vi "FileExplorer.vi"() -> ()   [LabVIEW 2010]
panel:
  in  "löschen":bool
  out "Numeric":i32
  out "error out 2":errorcluster
  out "filenames":string[](array[string])
  out "folder names":string[](array[string])
  out "error out":errorcluster
  in  "path":path
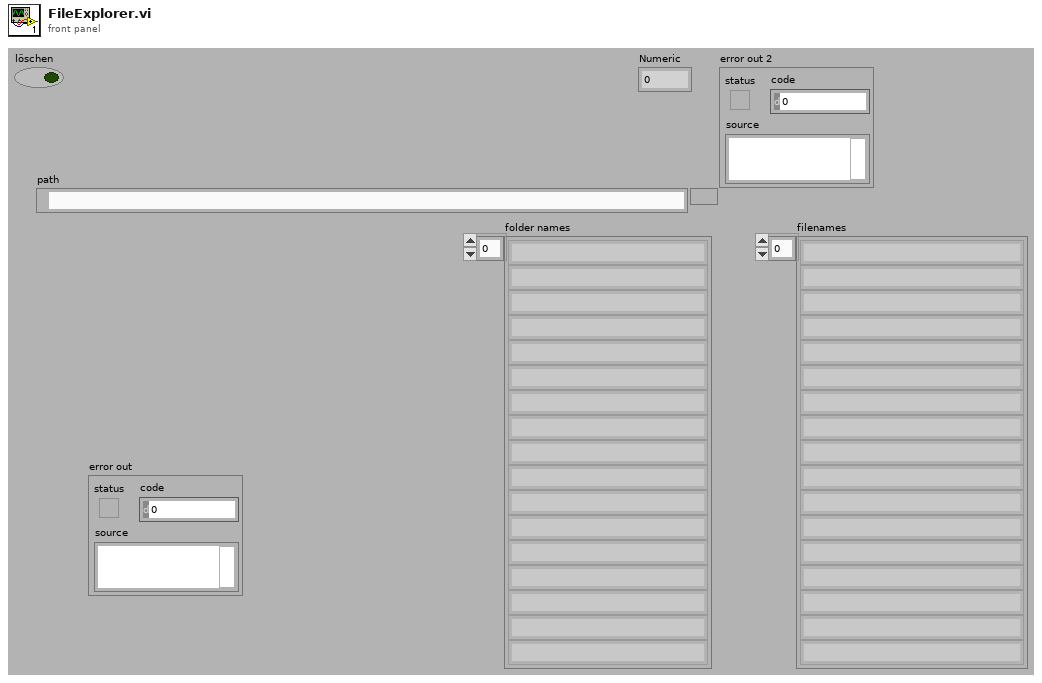
[diagram p1: front panel]
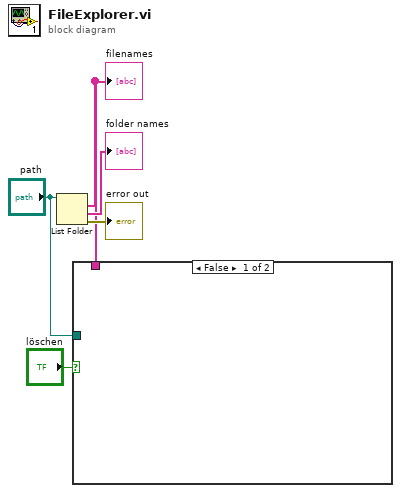
[diagram p0: block diagram]
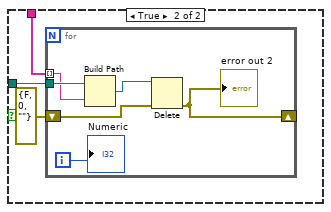
[diagram p2: hidden frame]
diagram:
  n1 = List Folder(path="path") -> (filenames=w3:string[], folder names=→"folder names":string[], error out=→"error out":errorcluster)  [unwired: 3 in, 1 out]
  "filenames" <- w3
  n2 = case shown="False" "löschen" {
    tunnel: w3 -> [_ w8]
    tunnel: "path" -> [_ w7]
    frame False {
    }
    frame True {
      n3 = for {
        tunnel: w8 -> [w13] mode=indexing
        tunnel: w7 -> [w14]
        shift-right: [w11] -> _
        shift-left: errorcluster {"status"=FALSE, "code"=0, "source"=""} ("error out") -> [w10]
        i -> [w9]
        n4 = Build Path(base path=w14, name or relative path=w13) -> (appended path=w12:path)
        n5 = Delete(path (use dialog)=w12, error in=w10) -> (error out=w11:errorcluster)  [unwired: 3 in, 2 out]
        "error out 2" <- w11
        "Numeric" <- w9
      }
    }
  }
